vi "Scale I32 to U8.vi"(5 "Input":i32) -> (2 "Output":u8)   [LabVIEW 2015]
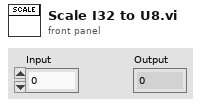
[diagram p1: front panel]
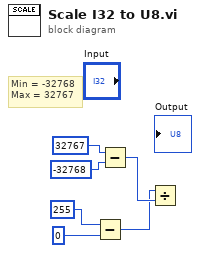
[diagram p0: block diagram]
diagram:
  # "Min = -32768\nMax = 32767"
  n1 = Subtract(x=255, y=0) -> (x-y=w1:i32)
  n2 = Subtract(x=32767, y=-32768) -> (x-y=w2:i32)
  n3 = Divide(x=w1, y=w2) -> ()  [unwired: 1 out]
